vi "get_angle.vi"(1 "CY":dbl, 2 "CX":dbl, 3 "DY":dbl, 4 "DX":dbl) -> (0 "ans":dbl)   [LabVIEW 2013]
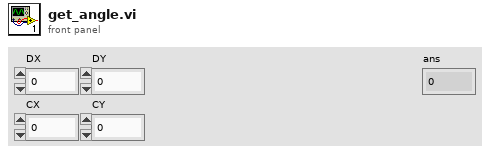
[diagram p1: front panel]
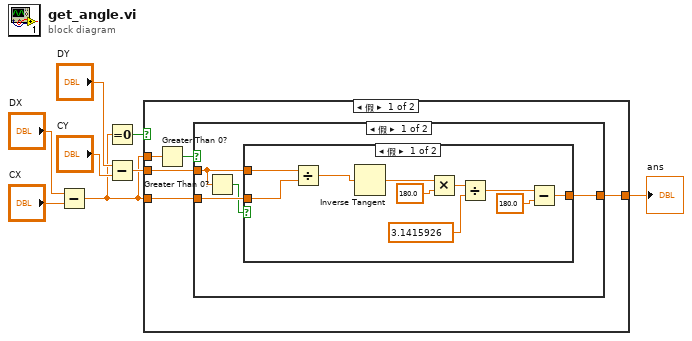
[diagram p0: block diagram]
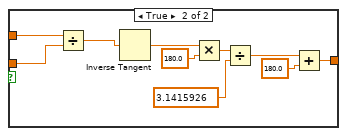
[diagram p2: hidden frame]
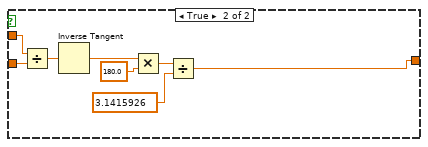
[diagram p3: hidden frame]
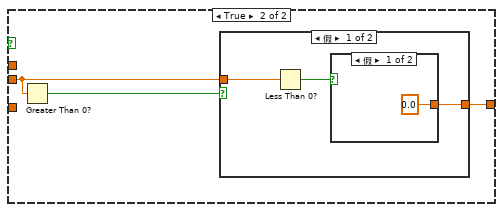
[diagram p4: hidden frame]
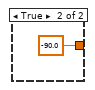
[diagram p5: hidden frame]
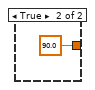
[diagram p6: hidden frame]
diagram:
  n1 = Subtract(x="DX", y="CX") -> (x-y=w1:dbl)
  n2 = Equal To 0?(x=w1) -> (x = 0?=w4:bool)
  n3 = Subtract(x="DY", y="CY") -> (x-y=w3:dbl)
  n4 = case shown="假" w4 {
    tunnel: w3 -> [w13 w46]
    tunnel: w1 -> [w12 _]
    tunnel: [w11 w47] -> w2
    tunnel: w1 -> [w9 _]
    frame False {
      n5 = Greater Than 0?(x=w9) -> (x > 0?=w10:bool)
      n6 = case shown="假" w10 {
        tunnel: w13 -> [w15 w44]
        tunnel: w12 -> [w17 w43]
        tunnel: [w14 w38] -> w11
        frame False {
          n7 = Greater Than 0?(x=w15) -> (x > 0?=w16:bool)
          n8 = case shown="假" w16 {
            tunnel: w15 -> [w19 w32]
            tunnel: w17 -> [w18 w31]
            tunnel: [w22 w28] -> w14
            frame False {
              n9 = Divide(x=w19, y=w18) -> (x/y=w23:dbl)
              n10 = Inverse Tangent(1:w23) -> (0:w24:dbl)
              n11 = Multiply(x=w24, y=180.0) -> (x*y=w26:dbl)
              n12 = Divide(x=w26, y=3.1415926) -> (x/y=w20:dbl)
              n13 = Subtract(x=w20, y=180.0) -> (x-y=w22:dbl)
            }
            frame True {
              n14 = Divide(x=w32, y=w31) -> (x/y=w37:dbl)
              n15 = Inverse Tangent(1:w37) -> (0:w36:dbl)
              n16 = Multiply(x=w36, y=180.0) -> (x*y=w34:dbl)
              n17 = Divide(x=w34, y=3.1415926) -> (x/y=w30:dbl)
              n18 = Add(x=w30, y=180.0) -> (x+y=w28:dbl)
            }
          }
        }
        frame True {
          n19 = Divide(x=w44, y=w43) -> (x/y=w45:dbl)
          n20 = Inverse Tangent(1:w45) -> (0:w42:dbl)
          n21 = Multiply(x=w42, y=180.0) -> (x*y=w40:dbl)
          n22 = Divide(x=w40, y=3.1415926) -> (x/y=w38:dbl)
        }
      }
    }
    frame True {
      n23 = Greater Than 0?(x=w46) -> (x > 0?=w48:bool)
      n24 = case shown="假" w48 {
        tunnel: [w51 90.0] -> w47
        tunnel: w46 -> [w49 _]
        frame False {
          n25 = Less Than 0?(x=w49) -> (x < 0?=w50:bool)
          n26 = case shown="假" w50 {
            tunnel: [0.0 -90.0] -> w51
            frame False {
            }
            frame True {
            }
          }
        }
        frame True {
        }
      }
    }
  }
  "ans" <- w2
